vi "ConfigMultiPointLowLevel.vi"(4 "eTriggerSource":u16, 6 "eSampleTrigger":u16, 7 "iTriggerCount":i32, 8 "error in (no error)":errorcluster, 9 "dSampleInterval":dbl, 10 "iSampleCount":i32, 11 "HP3458 VISA resource name":refnum<visa-resource-name>) -> (0 "error out":errorcluster)   [LabVIEW 2014, in "SamplerPlugins.lvlib" / "HP3458aDMM.lvclass"]
uses:
  HP3458aDMM.lvclass
  <vilib>/Utility/error.llb/Error Cluster From Error Code.vi
  <vilib>/ErrorRing/Error Ring.xnode
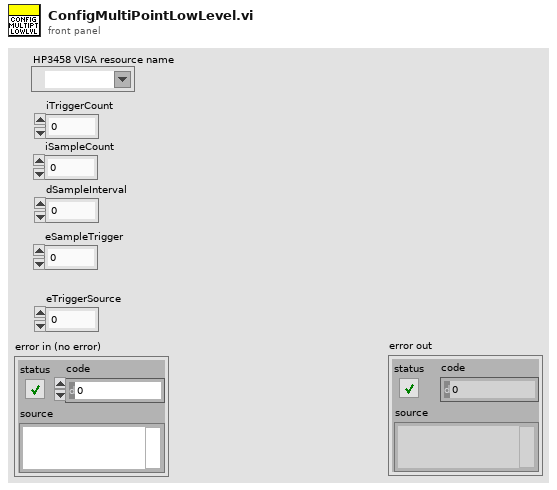
[diagram p1: front panel]
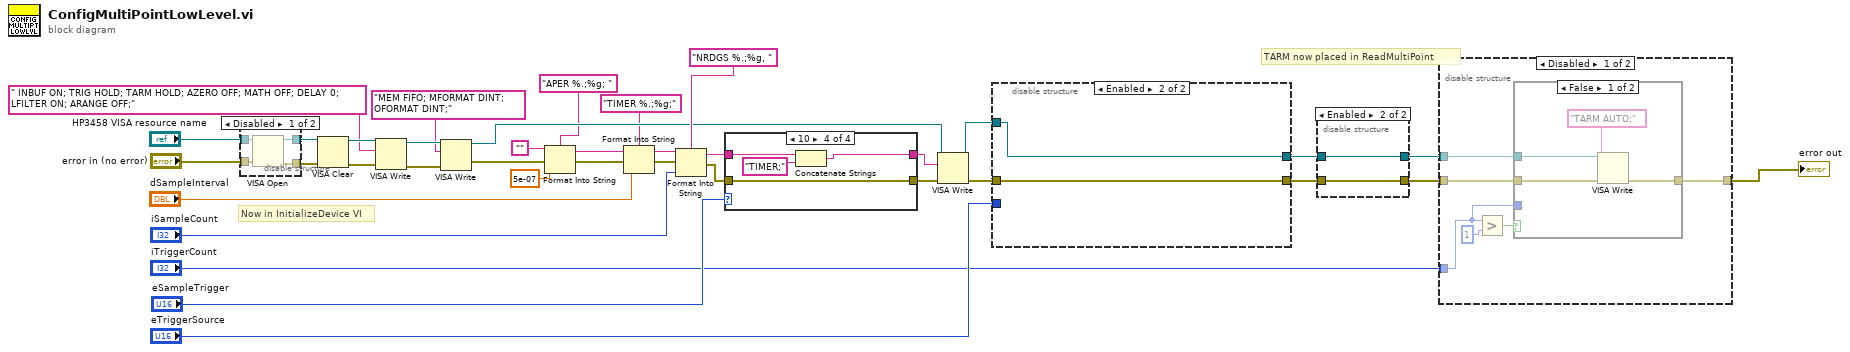
[diagram p0: block diagram]
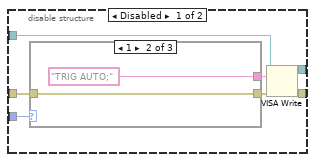
[diagram p2: hidden frame]
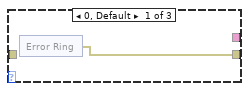
[diagram p3: hidden frame]
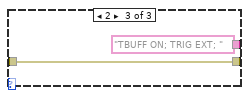
[diagram p4: hidden frame]
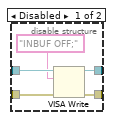
[diagram p5: hidden frame]
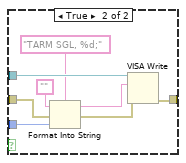
[diagram p7: hidden frame]
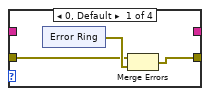
[diagram p9: hidden frame]
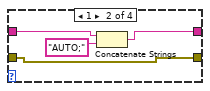
[diagram p10: hidden frame]
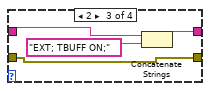
[diagram p11: hidden frame]
diagram:
  # "Now in InitializeDevice VI"
  # "TARM now placed in ReadMultiPoint"
  n1 = disable-structure shown="Disabled" {
    disable-tunnel: [w41 w43] -> w33
    disable-tunnel: [w40 w42] -> w32
    disable-tunnel: "HP3458 VISA resource name" -> [w39 w43]
    disable-tunnel: "error in (no error)" -> [w38 w42]
    frame Disabled {
      n2 = VISA Open(error in (no error)=w38, VISA resource name=w39) -> (VISA resource name=w41:refnum<visa-resource-name>, error out=w40:errorcluster)  [unwired: 3 in]
    }
    frame Enabled {
    }
  }
  n3 = VISA Clear(VISA resource name=w33, error in (no error)=w32) -> (VISA resource name out=w34:refnum<visa-resource-name>, error out=w35:errorcluster)
  n4 = VISA Write(VISA resource name=w34, write buffer=" INBUF ON; TRIG HOLD; TARM HOLD; AZERO OFF; MATH OFF; DELAY 0; LFILTER ON; ARANGE OFF;" ("string"), error in (no error)=w35) -> (VISA resource name out=w36:refnum<visa-resource-name>, error out=w37:errorcluster)  [unwired: 1 out]
  n5 = VISA Write(VISA resource name=w36, write buffer="MEM FIFO; MFORMAT DINT; OFORMAT DINT;", error in (no error)=w37) -> (VISA resource name out=w24:refnum<visa-resource-name>, error out=w27:errorcluster)  [unwired: 1 out]
  n6 = Format Into String(format string="APER %.;%g; " ("string"), initial string="", error in=w27, 5e-07 ("input 1")) -> (resulting string=w18:string, error out=w21:errorcluster)
  n7 = Format Into String(format string="TIMER %.;%g;", initial string=w18, error in=w21, "dSampleInterval") -> (resulting string=w17:string, error out=w20:errorcluster)
  n8 = Format Into String(format string="NRDGS %.;%g, ", initial string=w17, error in=w20, "iSampleCount") -> (resulting string=w15:string, error out=w14:errorcluster)
  n9 = case shown="10" "eSampleTrigger" {
    tunnel: w15 -> [_ w54 w58 w63]
    tunnel: [_ w53 w57 w61] -> w8
    tunnel: w14 -> [w45 w52 w56 w60]
    tunnel: [w44 w52 w56 w60] -> w13
    frame 0, Default {
      n10 = xnode "Error Ring"() -> ("error out"=w46:errorcluster)
      n11 = Merge Errors(w45, w46) -> (w44:errorcluster)
    }
    frame 1 {
      n12 = Concatenate Strings(w54, "AUTO;" ("string")) -> (w53:string)
    }
    frame 2 {
      n13 = Concatenate Strings(w58, "EXT; TBUFF ON;" ("string")) -> (w57:string)
    }
    frame 10 {
      n14 = Concatenate Strings(w63, "TIMER;" ("string")) -> (w61:string)
    }
  }
  n15 = VISA Write(VISA resource name=w24, write buffer=w8, error in (no error)=w13) -> (VISA resource name out=w11:refnum<visa-resource-name>, error out=w10:errorcluster)  [unwired: 1 out]
  n16 = disable-structure shown="Enabled" {
    disable-tunnel: w11 -> [w70 w81]
    disable-tunnel: w10 -> [w69 w82]
    disable-tunnel: "eTriggerSource" -> [w67 _]
    disable-tunnel: [w65 w81] -> w5
    disable-tunnel: [w64 w82] -> w4
    frame Disabled {
      n17 = case shown="1" w67 {
        tunnel: w69 -> [_ w77 w80]
        tunnel: [w71 w77 w80] -> w68
        tunnel: [_ "TRIG AUTO;" ("write buffer") "TBUFF ON; TRIG EXT; " ("write buffer")] -> w66
        frame 0, Default {
          n18 = xnode "Error Ring"() -> ("error out"=w71:errorcluster)
        }
        frame 1 {
        }
        frame 2 {
        }
      }
      n19 = VISA Write(VISA resource name=w70, write buffer=w66, error in (no error)=w68) -> (VISA resource name out=w65:refnum<visa-resource-name>, error out=w64:errorcluster)  [unwired: 1 out]
    }
    frame Enabled {
    }
  }
  n20 = disable-structure shown="Enabled" {
    disable-tunnel: w5 -> [w87 w89]
    disable-tunnel: w4 -> [w86 w88]
    disable-tunnel: [w85 w89] -> w3
    disable-tunnel: [w84 w88] -> w2
    frame Disabled {
      n21 = VISA Write(VISA resource name=w87, write buffer="INBUF OFF;", error in (no error)=w86) -> (VISA resource name out=w85:refnum<visa-resource-name>, error out=w84:errorcluster)  [unwired: 1 out]
    }
    frame Enabled {
    }
  }
  n22 = disable-structure shown="Disabled" {
    disable-tunnel: w3 -> [w94 _]
    disable-tunnel: w2 -> [w93 w108]
    disable-tunnel: [w92 w108] -> w7
    disable-tunnel: "iTriggerCount" -> [w90 _]
    frame Disabled {
      n23 = Greater?(x=w90, y=1) -> (0:w91:bool)
      n24 = case shown="False" w91 {
        tunnel: w94 -> [w98 w106]
        tunnel: w93 -> [w97 w101]
        tunnel: [w96 w107] -> w92
        tunnel: w90 -> [_ w105]
        frame False {
          n25 = VISA Write(VISA resource name=w98, write buffer="TARM AUTO;", error in (no error)=w97) -> (error out=w96:errorcluster)  [unwired: 2 out]
        }
        frame True {
          n26 = Format Into String(format string="TARM SGL, %d;", initial string="", error in=w101, w105) -> (resulting string=w102:string, error out=w100:errorcluster)
          n27 = VISA Write(VISA resource name=w106, write buffer=w102, error in (no error)=w100) -> (error out=w107:errorcluster)  [unwired: 2 out]
        }
      }
    }
    frame Enabled {
    }
  }
  "error out" <- w7
